vi "例程03-程序结构.vi"() -> ()   [LabVIEW 2016]
panel:
  out "单击次数":dbl
  in  "事件结构测试":bool
  out "Numeric":i32
  out "floor(x/y)":i32
  out "x-y*floor(x/y)":i32
  out "Boolean":bool
  out "波形图表 2":dbl(graph)
  out "while循环计数器":i32
  out "for循环计数器":i32
  out "波形图表":dbl(graph)
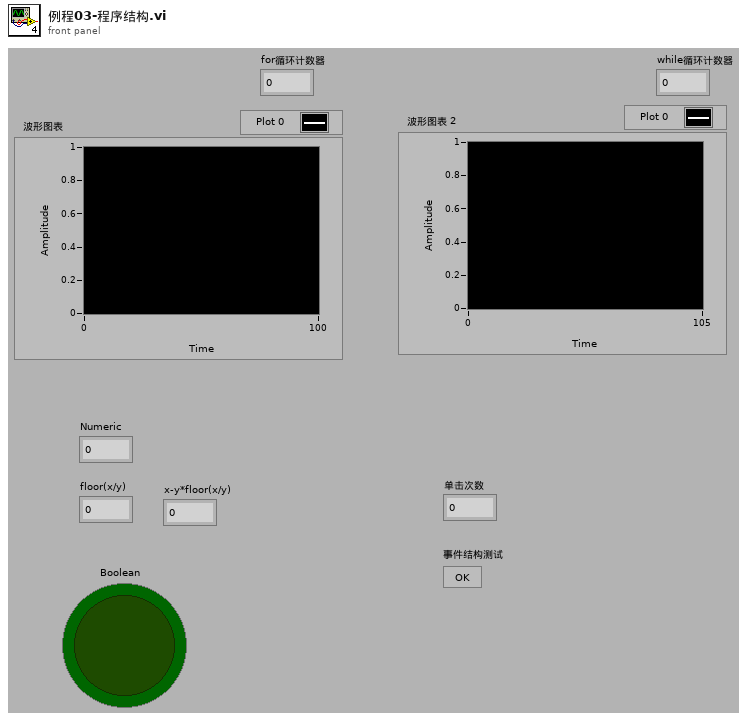
[diagram p1: front panel]
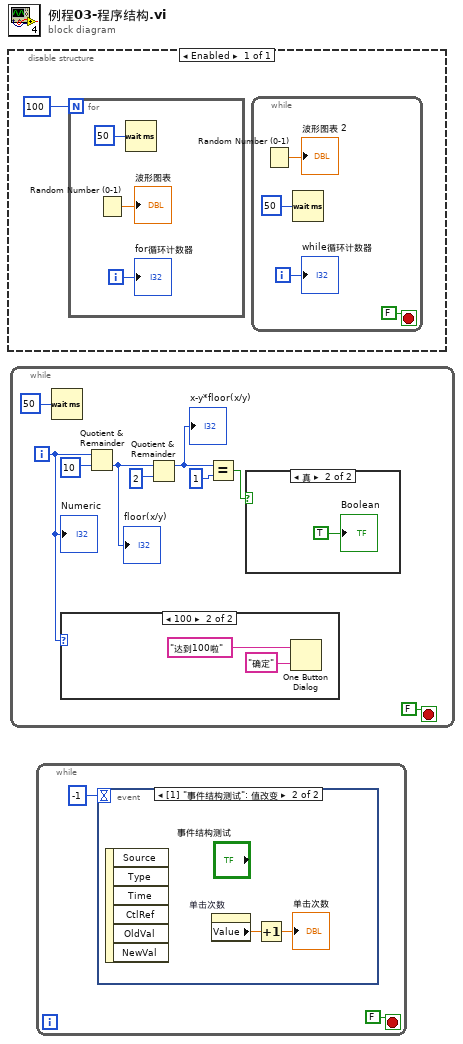
[diagram p0: block diagram]
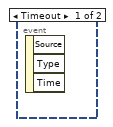
[diagram p2: hidden frame]
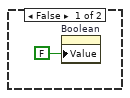
[diagram p4: hidden frame]
diagram:
  n1 = disable-structure shown="Enabled" {
    frame Enabled {
      n2 = for {
        N: 100 -> [_]
        i -> [w6]
        n3 = Random Number (0-1)() -> (number: 0 to 1=→"波形图表":dbl)
        n4 = Wait (ms)(milliseconds to wait=u32 50) -> ()  [unwired: 1 out]
        "for循环计数器" <- w6
      }
      n5 = while {
        i -> [w5]
        stop <- FALSE stop-if-true
        n6 = Random Number (0-1)() -> (number: 0 to 1=→"波形图表 2":dbl)
        n7 = Wait (ms)(milliseconds to wait=u32 50) -> ()  [unwired: 1 out]
        "while循环计数器" <- w5
      }
    }
  }
  n8 = while {
    i -> [w9]
    stop <- FALSE stop-if-true
    n9 = Wait (ms)(milliseconds to wait=u32 50) -> ()  [unwired: 1 out]
    n10 = case shown="100" w9 {
      frame 0, Default {
      }
      frame 100 {
        n11 = One Button Dialog(message="达到100啦", button name ("OK")="确定") -> ()  [unwired: 1 out]
      }
    }
    n12 = Quotient & Remainder(x=w9, y=10) -> (floor(x/y)=w10:i32)  [unwired: 1 out]
    "floor(x/y)" <- w10
    n13 = Quotient & Remainder(x=w10, y=2 ("x")) -> (x-y*floor(x/y)=w12:i32)  [unwired: 1 out]
    "x-y*floor(x/y)" <- w12
    n14 = Equal?(x=w12, y=1) -> (x = y?=w15:bool)
    n15 = case shown="真" w15 {
      frame False {
        n16 = property on="Boolean" class="Bool (严格)"("Value"=FALSE ("Boolean")) -> ()  [unwired: 2 in, 2 out]
      }
      frame True {
        "Boolean" <- TRUE ("Boolean")
      }
    }
    "Numeric" <- w9
  }
  n17 = while {
    stop <- FALSE stop-if-true
    n18 = event shown="[1] \"事件结构测试\": 值改变" {
      selector: _ -> [_ _]
      dyn-events: _ -> [_ _]
      timeout: -1 -> [_ _]
      event Timeout {
        n19 = event-data() -> ()  [unwired: 1 in, 3 out]
      }
      event "事件结构测试": Value Change {
        n20 = event-data() -> ()  [unwired: 1 in, 6 out]
        n21 = property on="单击次数" class="DigNum (严格)"() -> ("Value"=w25:dbl)  [unwired: 2 in, 2 out]
        n22 = Increment(x=w25) -> (x+1=→"单击次数":dbl)
      }
    }
  }
